vi "Negate Complex Number.vi"(1 "ComplexNumber in":refnum<class "ComplexNumberStatic.lvclass">) -> (0 "ComplexNumber out":refnum<class "ComplexNumberStatic.lvclass">)   [LabVIEW 2014]
uses:
  <vilib>/LabVIEW Universal Transcriptor/LabVIEW for Arduino Complex Numbers Static/ComplexNumberStatic.lvclass
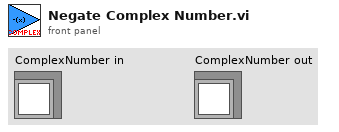
[diagram p1: front panel]
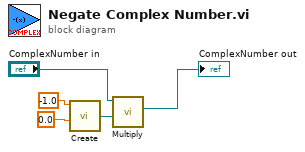
[diagram p0: block diagram]
diagram:
  n1 = call <vilib>:"Create.vi"("Imag"=0.0, "Real"=-1.0) -> ("ComplexNumber"=w5:refnum<class "ComplexNumberStatic.lvclass">)  [unwired: 3 in, 1 out]
  n2 = call <vilib>:"Multiply.vi"("B"=w5, "A"="ComplexNumber in") -> ("A*B"=→"ComplexNumber out":refnum<class "ComplexNumberStatic.lvclass">)  [unwired: 8 in, 1 out]
